vi "AnalysatorAuswahl befuellen.vi"(8 "error in (no error)":errorcluster caption="Fehler (Eingang, kein Fehler)", 10 "Analysatoren":string[](array[string]), 11 "Analysator Definition (Eingang)":refnum<vi>) -> (0 "error out":errorcluster caption="Fehler (Ausgang)")   [LabVIEW 2020, in "System Einstellungen V2.lvlib"]
uses:
  System Einstellungen V2.lvlib
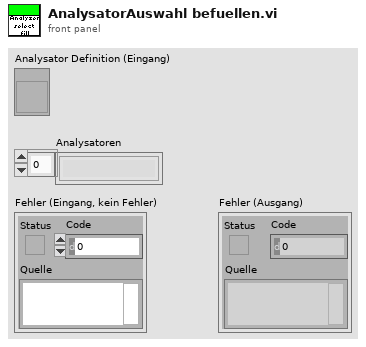
[diagram p1: front panel]
types:
  T1 = cluster{"Analysator":string, "Analysator":string}
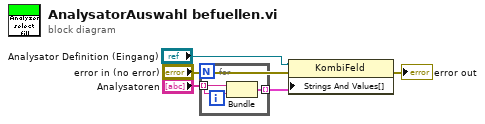
[diagram p0: block diagram]
diagram:
  n1 = for {
    tunnel: [w7] -> w2 mode=indexing
    tunnel: "Analysatoren" -> [w6] mode=indexing
    n2 = Bundle("Analysator"=w6, "Analysator"=w6) -> (w7:T1)  [unwired: 1 in]
  }
  n3 = property class="KombiFeld"(reference="Analysator Definition (Eingang)", error in="error in (no error)", "Strings And Values[]"=w2) -> (error out=→"error out":errorcluster)  [unwired: 1 out]
